vi "Range Index.vi"(1 "Index":i32, 2 "Size":i32) -> (3 "Index Out Out":i32)   [LabVIEW 2020, in "Absolute_Pointer.lvclass"]
uses:
  Absolute_Pointer.lvclass
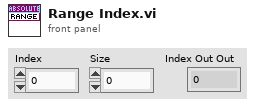
[diagram p1: front panel]
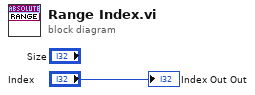
[diagram p0: block diagram]
diagram:
  "Index Out Out" <- "Index"
